vi "chess draw.vi"(1 "rect":T1, 2 "Chess":i32, 3 "Color":i32, 4 "In Pic":picture) -> (0 "Out Pic":picture)   [LabVIEW 2009]
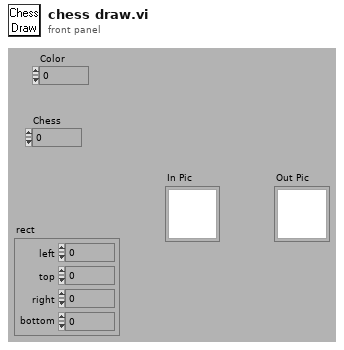
[diagram p1: front panel]
types:
  T1 = cluster{"left":i16, "top":i16, "right":i16, "bottom":i16}
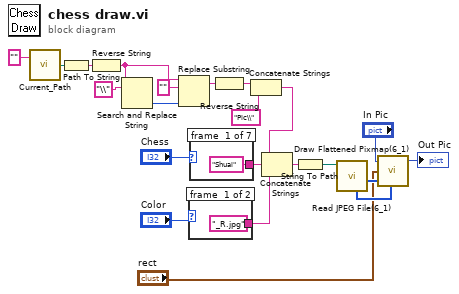
[diagram p0: block diagram]
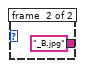
[diagram p2: hidden frame]
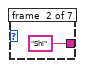
[diagram p3: hidden frame]
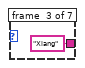
[diagram p4: hidden frame]
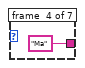
[diagram p5: hidden frame]
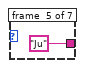
[diagram p6: hidden frame]
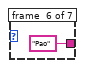
[diagram p7: hidden frame]
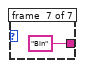
[diagram p8: hidden frame]
diagram:
  n1 = call "Current_Path.vi"("Dir Or File Name"="") -> ("Dir or File In Current Path"=w10:path)  [unwired: 1 in]
  n2 = Path To String(path=w10) -> (string=w7:string)
  n3 = Reverse String(1:w7) -> (0:w5:string)
  n4 = Search and Replace String(input string=w5, search string="\\") -> (offset past replacement=w3:i32)  [unwired: 1 in, 8 out]
  n5 = Replace Substring(2:w3, 4:"" ("substring (\"\")"), 5:w5) -> (1:w2:string)  [unwired: 2 out]
  n6 = case shown="1, Default" "Color" {
    tunnel: ["_R.jpg" "_B.jpg"] -> w14
    frame #0 {
    }
    frame #1 {
    }
  }
  n7 = case shown="6" "Chess" {
    tunnel: ["Shuai" "Shi" "Xiang" "Ma" "Ju" "Pao" "Bin"] -> w15
    frame #0 {
    }
    frame #1 {
    }
    frame #2 {
    }
    frame #3 {
    }
    frame #4 {
    }
    frame #5 {
    }
    frame #6 {
    }
  }
  n8 = Reverse String(1:w2) -> (0:w1:string)
  n9 = Concatenate Strings(w1, "Pic\\" ("Substring")) -> (w8:string)
  n10 = Concatenate Strings(w8, w15, w14) -> (w13:string)
  n11 = String To Path(string=w13) -> (path=w12:path)
  n12 = call <vilib>:"Read JPEG File(6_1).vi"("path to JPEG file"=w12) -> ("flattened image data"=w21:u8[], "colorTable"=w22:u32[])  [unwired: 1 in, 8 out]
  n13 = call <vilib>:"Draw Flattened Pixmap(6_1).vi"("picture"="In Pic", "rect"="rect", "flattened pixmap data"=w21, "color table"=w22) -> ("new picture"=→"Out Pic":picture)  [unwired: 1 in, 4 out]
